vi "Assign ID.vi"(11 "Topic in":refnum<class "Topic.lvclass">) -> (3 "Topic out":refnum<class "Topic.lvclass">)   [LabVIEW 2015, in "Mediator.lvlib" / "Topic.lvclass"]
uses:
  Topic.lvclass
  Topic.lvclass/Topic.ctl
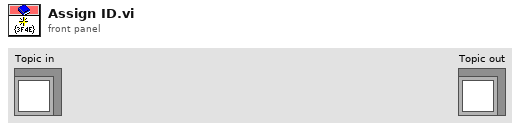
[diagram p1: front panel]
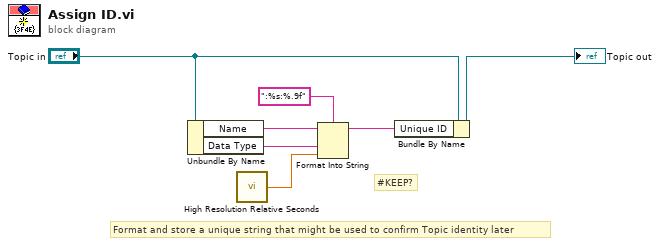
[diagram p0: block diagram]
diagram:
  # "#KEEP?"
  # "Format and store a unique string that might be used to confirm Topic identity later"
  n1 = Unbundle By Name("Topic in") -> ("Name"=w5:string, "Data Type"=w4:string)
  n2 = call <vilib>:"High Resolution Relative Seconds.vi"() -> ("relative seconds"=w3:dbl)
  n3 = Format Into String(format string=":%s:%.9f", initial string=w5, w4, w3) -> (resulting string=w2:string)  [unwired: 1 in, 1 out]
  n4 = Bundle By Name(cluster="Topic in", "Unique ID"=w2) -> (→"Topic out":refnum<class "Topic.lvclass">)
